vi "fpga_all_example.vi"() -> ()   [LabVIEW 2018]
uses:
  <vilib>/Platform/TimedLoop/XDataNode/timing_clust.ctl
  <vilib>/Platform/TimedLoop/XDataNode/nitl_modes.ctl
  <vilib>/Platform/TimedLoop/XDataNode/wakeup.ctl
  <vilib>/rvi/Emulation/niFpgaGetClockAttributes.vi
  <vilib>/rvi/Emulation/niFpgaSctlEmulationGetInTimedLoop.vi
  <vilib>/rvi/Emulation/niFpgaEmulationReportErrorSimple.vi
  <vilib>/rvi/eio/common/nirviEmuTemplateMethod_errors.vi
  <vilib>/rvi/Emulation/niFpgaCriticalErrorInLSC.vi
  <vilib>/rvi/Emulation/niFpgaProcessEmulError.vi
  lib/Cast-EPICS/cast u64 to u-64-64.vi
  lib/Cast-EPICS/cast u-64-64 to u64.vi
  lib/Cast-EPICS/cast u64 to u-64-0.vi
  lib/Cast-EPICS/cast u-64-0 to u64.vi
  lib/Cast-EPICS/cast u64 to u-64-32.vi
  lib/Cast-EPICS/cast u-64-32 to u64.vi
  lib/Cast-EPICS/cast u64 to s-64-0.vi
  lib/Cast-EPICS/cast s-64-0 to u64.vi
  lib/Cast-EPICS/cast u64 to s-64-64.vi
  lib/Cast-EPICS/cast s-64-64 to u64.vi
  lib/Cast-EPICS/cast u64 to s-64-32.vi
  lib/Cast-EPICS/cast s-64-32 to u64.vi
  <vilib>/eio/EIONode/EIONode.xnode
  <vilib>/Platform/TimedLoop/XDataNode/XDataNode.xnode
  <vilib>/Platform/TimedLoop/XDataNode/XDNodeRunTimeDep.lvlib
  lib/Scaler-EPICS/scaler.lvlib
  lib/Cast-EPICS/fixedpoint-cast.lvlib
panel:
  out "fxp_AnalogOutput3_SCALER2":u64
  out "fxp_AnalogOutput2_SCALER2":u64
  out "fxp_AnalogOutput1_SCALER2":u64
  out "fxp_AnalogOutput0_SCALER2":u64
  in  "fxp_ShiftLeft_SCALER2":u64
  out "fixedpoint_i 1":fxp<+,64,64> format="%.20f"
  out "aifxp 1":u64
  out "fixedpoint_i 2":fxp<+,64,0> format="%#_20g"
  out "aifxp 2":u64
  out "fixedpoint_i 3":fxp<+,64,32> format="%#_20g"
  out "aifxp 3":u64
  out "fixedpoint_i 4":fxp<+/-,64,0> format="%#_20g"
  out "aifxp 4":u64
  out "fixedpoint_i 5":fxp<+/-,64,64> format="%.20f"
  out "aifxp 5":u64
  out "fixedpoint_i 6":fxp<+/-,64,32> format="%#_20g"
  out "aifxp 6":u64
  in  "aofxp 1":u64
  in  "aofxp 2":u64
  in  "aofxp 3":u64
  in  "aofxp 4":u64
  in  "aofxp 5":u64
  in  "aofxp 6":u64
  in  "waveform_u32 2":u32[](array[numeric])=[0, 0, 0]
  out "waveform_u32":u32[](array[numeric])
  out "waveform_u64 2":u64[](array[numeric])
  out "waveform_sgl 2":sgl[](array[numeric]) format="%.2f"
  in  "waveform_u64":u64[](array[numeric])=[0, 0, 0]
  in  "waveform_sgl":sgl[](array[numeric])=[0.0, 0.0, 0.0]
  out "waveform_u16 2":u16[](array[numeric])
  in  "waveform_u16":u16[](array[numeric])=[0, 0, 0]
  out "waveform_u8 2":u8[](array[numeric])
  in  "waveform_u8":u8[](array[numeric])=[0, 0, 0]
  out "waveform_i8 2":i8[](array[numeric])
  in  "waveform_i8":i8[](array[numeric])=[0, 0, 0]
  out "waveform_i16 2":i16[](array[numeric])
  in  "waveform_i16":i16[](array[numeric])=[0, 0, 0]
  out "waveform_i32 2":i32[](array[numeric])
  in  "waveform_i32":i32[](array[numeric])=[0, 0, 0]
  out "waveform_i64 2":i64[](array[numeric])
  in  "waveform_i64":i64[](array[numeric])=[0, 0, 0]
  out "Looptime":u32
  out "AnalogInputs_SCALER2":fxp<+/-,20,5>[](array[numeric])
  in  "PresetValues_SCALER2":u32[](array[numeric])=[0, 0, 0, 0, 0]
  in  "Gate_SCALER2":bool[](array[boolean])=[FALSE, FALSE, FALSE, FALSE, FALSE]
  in  "OneShot_SCALER2":bool
  in  "Enable_SCALER2":bool
  out "Counter_SCALER2":u32[](array[numeric])
  out "Done_SCALER2":bool
  in  "SampleAnalog_SCALER2":bool
  in  "OneShot_SCALER1":bool
  in  "Enable_SCALER1":bool
  in  "Gate_SCALER1":bool[](array[boolean])=[FALSE, FALSE]
  out "Done_SCALER1":bool
  out "Counter_SCALER1":u32[](array[numeric])
  in  "PresetValues_SCALER1":u32[](array[numeric])=[0, 0]
  in  "Pulse_SCALER1":bool[](array[boolean])=[FALSE]
  in  "Mod3/DIO31":bool
  in  "Mod3/DIO30":bool
  in  "Mod3/DIO29":bool
  in  "Mod3/DIO28":bool
  in  "Mod3/DIO27":bool
  in  "Mod3/DIO26":bool
  in  "Mod3/DIO25":bool
  in  "Mod3/DIO24":bool
  in  "Mod3/DIO23":bool
  in  "Mod3/DIO22":bool
  in  "Mod3/DIO21":bool
  in  "Mod3/DIO20":bool
  in  "Mod3/DIO19":bool
  in  "Mod3/DIO18":bool
  in  "Mod3/DIO17":bool
  in  "Mod3/DIO16":bool
  in  "Mod2/DIO0":bool
  in  "Mod2/DIO1":bool
  in  "Mod2/DIO2":bool
  in  "Mod2/DIO3":bool
  in  "Mod1/DIO0":bool
  in  "Mod1/DIO1":bool
  in  "Mod1/DIO2":bool
  in  "Mod1/DIO3":bool
  out "BI":u64
  out "aiMod4/AI3":sgl format="%#_64g"
  out "aiMod4/AI2":sgl format="%#_64g"
  out "aiMod4/AI1":sgl format="%#_64g"
  out "aiMod4/AI0":sgl format="%#_64g"
  in  "aoMod5/AO0":sgl format="%#_64g"
  in  "aoMod5/AO1":sgl format="%#_64g"
  in  "aoMod5/AO2":sgl format="%#_64g"
  in  "aoMod5/AO3":sgl format="%#_64g"
  out "aiMod7/AI3":sgl format="%#_64g"
  out "aiMod7/AI2":sgl format="%#_64g"
  out "aiMod7/AI1":sgl format="%#_64g"
  out "aiMod7/AI0":sgl format="%#_64g"
  out "aiMod8/AI0":sgl format="%#_64g"
  out "aiMod8/AI1":sgl format="%#_64g"
  out "aiMod8/AI2":sgl format="%#_64g"
  out "aiMod8/AI3":sgl format="%#_64g"
  # "Scalers"
  # "Binary outputs"
  # "Analog\nOutput"
  # "Binary\nInput"
  # "Analog Input"
  # "Fixedpoint controls and Indicators"
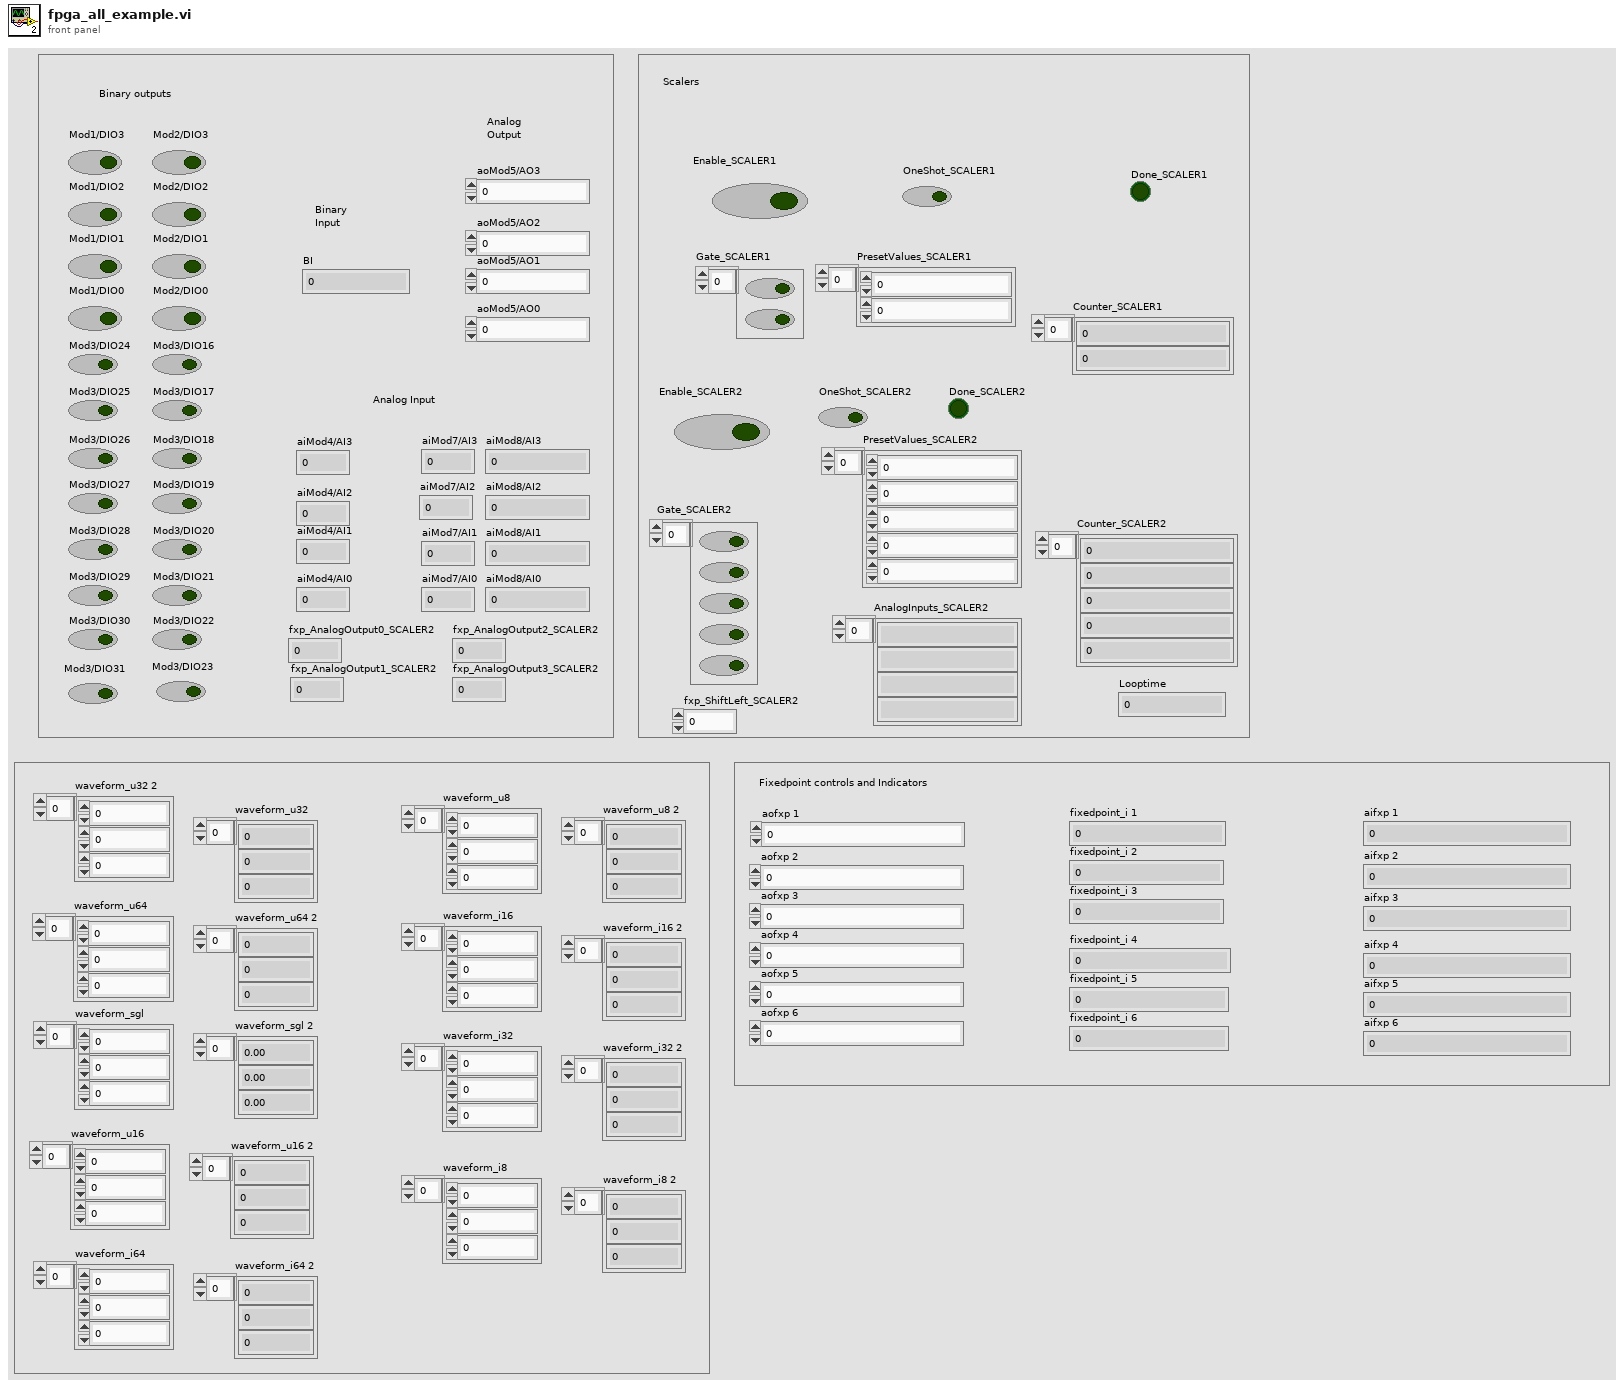
[diagram p1: front panel]
types:
  T1 = typedef "XDNodeRunTimeDep.lvlib/timing_clust.ctl" = cluster{"Expected End [f-1]":u64, "Actual End [f-1]":u64, "Finished Late? [f-1]":bool, "Expected End [i-1]":u64, "Actual End [i-1]":u64, "Finished Late? [i-1]":bool, "Expected Start [i]":u64, "Actual Start [i]":u64, "Expected Start [f]":u64, "Actual Start [f]":u64, "Source Name":string, "Structure Name":string, "Period":i64, "Deadline":i64, "Offset":i64, "Start":i64, "Priority":i32, "Timeout":i32, "Mode":T2, "Wakeup Reason":T3, "Error":errorcluster, "Source Type":string, "Secondary Source Type":string, "Global End Time":u64, "Global Start Time":u64, "Frame Duration":u64, "Iteration Duration":u64, "Assigned CPU":i32, "I/O Scan Engine Mode":u32}
  T2 = typedef "XDNodeRunTimeDep.lvlib/nitl_modes.ctl" = enum32{"No Change", "Process missed periods, maintain original phase", "Discard missed periods, maintain original phase", "Process missed periods, ignore original phase", "Discard missed periods, ignore original phase"}
  T3 = typedef "XDNodeRunTimeDep.lvlib/wakeup.ctl" = enum32{"Normal", "Aborted", "Asynchronous wakeup", "Timing source error", "Timed loop error", "Timeout"}
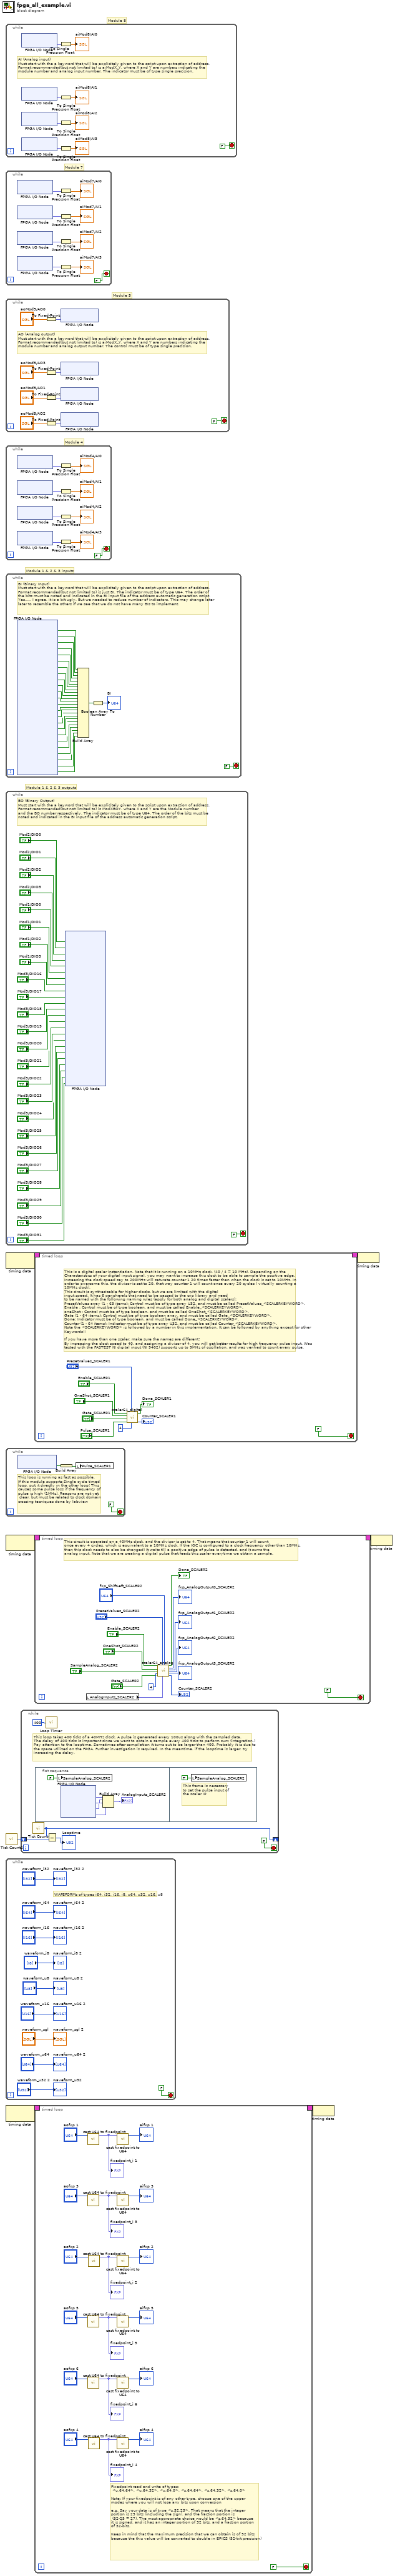
[diagram p0: block diagram]
diagram:
  # "Module 1 & 2 & 3 outputs"
  # "Module 1 & 2 & 3 inputs"
  # "Module 4"
  # "Module 5"
  # "Module 7"
  # "Module 8"
  n1 = while {
    stop <- FALSE stop-if-true
    # "AI (Analog input)\nMust start with the a keyword that will be explicitely given to the script upon extraction of address. \nFormat recommended(but not limited to) is aiModX_Y, where X and Y are numbers indicating the \nmodule number and analog input number. The indicator must be of type single precision."
    n2 = xnode "FPGA I/O Node"() -> ("Mod8/AI0"=w8:fxp<+/-,20,5>)  [unwired: 1 in, 1 out]
    n3 = xnode "FPGA I/O Node"() -> ("Mod8/AI1"=w12:fxp<+/-,20,5>)  [unwired: 1 in, 1 out]
    n4 = xnode "FPGA I/O Node"() -> ("Mod8/AI2"=w10:fxp<+/-,20,5>)  [unwired: 1 in, 1 out]
    n5 = xnode "FPGA I/O Node"() -> ("Mod8/AI3"=w15:fxp<+/-,20,5>)  [unwired: 1 in, 1 out]
    n6 = To Single Precision Float(number=w8) -> (single precision float=→"aiMod8/AI0":sgl)
    n7 = To Single Precision Float(number=w12) -> (single precision float=→"aiMod8/AI1":sgl)
    n8 = To Single Precision Float(number=w10) -> (single precision float=→"aiMod8/AI2":sgl)
    n9 = To Single Precision Float(number=w15) -> (single precision float=→"aiMod8/AI3":sgl)
  }
  n10 = while {
    stop <- FALSE stop-if-true
    n11 = xnode "FPGA I/O Node"() -> ("Mod7/AI0"=w22:fxp<+/-,20,5>)  [unwired: 1 in, 1 out]
    n12 = xnode "FPGA I/O Node"() -> ("Mod7/AI1"=w20:fxp<+/-,20,5>)  [unwired: 1 in, 1 out]
    n13 = xnode "FPGA I/O Node"() -> ("Mod7/AI2"=w18:fxp<+/-,20,5>)  [unwired: 1 in, 1 out]
    n14 = xnode "FPGA I/O Node"() -> ("Mod7/AI3"=w24:fxp<+/-,20,5>)  [unwired: 1 in, 1 out]
    n15 = To Single Precision Float(number=w22) -> (single precision float=→"aiMod7/AI0":sgl)
    n16 = To Single Precision Float(number=w20) -> (single precision float=→"aiMod7/AI1":sgl)
    n17 = To Single Precision Float(number=w18) -> (single precision float=→"aiMod7/AI2":sgl)
    n18 = To Single Precision Float(number=w24) -> (single precision float=→"aiMod7/AI3":sgl)
  }
  n19 = while {
    stop <- FALSE stop-if-true
    # "AO (Analog output)\nMust start with the a keyword that will be explicitely given to the script upon extraction of address. \nFormat recommended(but not limited to) is aiModX_Y, where X and Y are numbers indicating the \nmodule number and analog output number. The control must be of type single precision."
    n20 = To Fixed-Point(number="aoMod5/AO0") -> (fixed-point=w33:fxp<+/-,20,5>)  [unwired: 1 in]
    n21 = To Fixed-Point(number="aoMod5/AO3") -> (fixed-point=w30:fxp<+/-,20,5>)  [unwired: 1 in]
    n22 = To Fixed-Point(number="aoMod5/AO1") -> (fixed-point=w32:fxp<+/-,20,5>)  [unwired: 1 in]
    n23 = To Fixed-Point(number="aoMod5/AO2") -> (fixed-point=w31:fxp<+/-,20,5>)  [unwired: 1 in]
    n24 = xnode "FPGA I/O Node"("Mod5/AO0"=w33) -> ()  [unwired: 1 in, 1 out]
    n25 = xnode "FPGA I/O Node"("Mod5/AO3"=w30) -> ()  [unwired: 1 in, 1 out]
    n26 = xnode "FPGA I/O Node"("Mod5/AO1"=w32) -> ()  [unwired: 1 in, 1 out]
    n27 = xnode "FPGA I/O Node"("Mod5/AO2"=w31) -> ()  [unwired: 1 in, 1 out]
  }
  n28 = while {
    stop <- FALSE stop-if-true
    n29 = xnode "FPGA I/O Node"() -> ("Mod4/AI0"=w40:fxp<+/-,20,5>)  [unwired: 1 in, 1 out]
    n30 = xnode "FPGA I/O Node"() -> ("Mod4/AI1"=w38:fxp<+/-,20,5>)  [unwired: 1 in, 1 out]
    n31 = xnode "FPGA I/O Node"() -> ("Mod4/AI2"=w36:fxp<+/-,20,5>)  [unwired: 1 in, 1 out]
    n32 = xnode "FPGA I/O Node"() -> ("Mod4/AI3"=w42:fxp<+/-,20,5>)  [unwired: 1 in, 1 out]
    n33 = To Single Precision Float(number=w40) -> (single precision float=→"aiMod4/AI0":sgl)
    n34 = To Single Precision Float(number=w38) -> (single precision float=→"aiMod4/AI1":sgl)
    n35 = To Single Precision Float(number=w36) -> (single precision float=→"aiMod4/AI2":sgl)
    n36 = To Single Precision Float(number=w42) -> (single precision float=→"aiMod4/AI3":sgl)
  }
  n37 = while {
    stop <- FALSE stop-if-true
    # "BI (Binary Input)\nMust start with the a keyword that will be explicitely given to the script upon extraction of address. \nFormat recommended(but not limited to) is just BI. The indicator must be of type U64. The order of \nthe bits must be noted and indicated in the BI input file of the address automatic generation script.\nYes...., I agree, it is a bit ugly. But we needed to reduce number of indicators. This may change later\nlater to resemble the others if we see that we do not have many BIs to implement."
    n38 = xnode "FPGA I/O Node"() -> ("Mod3/DIO0"=w70:bool, "Mod3/DIO1"=w69:bool, "Mod3/DIO2"=w66:bool, "Mod3/DIO3"=w65:bool, "Mod3/DIO4"=w64:bool, "Mod3/DIO5"=w63:bool, "Mod3/DIO6"=w62:bool, "Mod3/DIO7"=w61:bool, "Mod3/DIO8"=w60:bool, "Mod3/DIO9"=w59:bool, "Mod3/DIO10"=w58:bool, "Mod3/DIO11"=w57:bool, "Mod3/DIO12"=w56:bool, "Mod3/DIO13"=w55:bool, "Mod3/DIO14"=w54:bool, "Mod3/DIO15"=w53:bool, "Mod1/DIO4"=w51:bool, "Mod1/DIO5"=w50:bool, "Mod1/DIO6"=w49:bool, "Mod1/DIO7"=w48:bool, "Mod2/DIO4"=w47:bool, "Mod2/DIO5"=w46:bool, "Mod2/DIO6"=w45:bool, "Mod2/DIO7"=w44:bool)  [unwired: 24 in, 24 out]
    n39 = Build Array(w70, w69, w66, w65, w64, w63, w62, w61, w60, w59, w58, w57, w56, w55, w54, w53, w51, w50, w49, w48, w47, w46, w45, w44) -> (w52:bool[])
    n40 = Boolean Array To Number(Boolean array=w52) -> (number=→"BI":u64)
  }
  n41 = while {
    stop <- FALSE stop-if-true
    # "BO (Binary Output)\nMust start with the a keyword that will be explicitely given to the script upon extraction of address. \nFormat recommended(but not limited to) is ModXBOY, where X and Y are the Module number \nand the BO number respectively. The indicator must be of type U64. The order of the bits must be \nnoted and indicated in the BI input file of the address automatic generation script."
    n42 = xnode "FPGA I/O Node"("Mod2/DIO0"="Mod2/DIO0", "Mod2/DIO1"="Mod2/DIO1", "Mod2/DIO2"="Mod2/DIO2", "Mod2/DIO3"="Mod2/DIO3", "Mod1/DIO0"="Mod1/DIO0", "Mod1/DIO1"="Mod1/DIO1", "Mod1/DIO2"="Mod1/DIO2", "Mod1/DIO3"="Mod1/DIO3", "Mod3/DIO16"="Mod3/DIO16", "Mod3/DIO17"="Mod3/DIO17", "Mod3/DIO18"="Mod3/DIO18", "Mod3/DIO19"="Mod3/DIO19", "Mod3/DIO20"="Mod3/DIO20", "Mod3/DIO21"="Mod3/DIO21", "Mod3/DIO22"="Mod3/DIO22", "Mod3/DIO23"="Mod3/DIO23", "Mod3/DIO24"="Mod3/DIO24", "Mod3/DIO25"="Mod3/DIO25", "Mod3/DIO26"="Mod3/DIO26", "Mod3/DIO27"="Mod3/DIO27", "Mod3/DIO28"="Mod3/DIO28", "Mod3/DIO29"="Mod3/DIO29", "Mod3/DIO30"="Mod3/DIO30", "Mod3/DIO31"="Mod3/DIO31") -> ()  [unwired: 24 in, 24 out]
  }
  n43 = node-c288() -> (w7:T1)  [unwired: 1 in]
  n44 = while {
    stop <- FALSE stop-if-true
    # "This loop is running as fast as possible. \nIf this module supports Single cycle timed\nloop, put it directly in the other loop! This\ncauses some pulse loss if the frequency of \npulse is high (1MHz). Reasons are not yet\n clear, but must be related to clock domain\ncrossing tecniques done by labview"
    n45 = xnode "FPGA I/O Node"() -> ("Mod2/DIO0"=w98:bool)  [unwired: 1 in, 1 out]
    n46 = Build Array(w98) -> (w97:bool[])
    n47 = local write "Pulse_SCALER1"(w97) -> ()
  }
  n48 = node-c288() -> (w5:T1)  [unwired: 1 in]
  n49 = call "Tick Count2"() -> ("Tick Count(Ticks)"=w3:u32)
  n50 = while {
    stop <- FALSE stop-if-true
    # "WAFEFORMs of types i64, i32, i16, i8, u64, u32, u16, u8"
    "waveform_u32" <- "waveform_u32 2"
    "waveform_u64 2" <- "waveform_u64"
    "waveform_sgl 2" <- "waveform_sgl"
    "waveform_u16 2" <- "waveform_u16"
    "waveform_u8 2" <- "waveform_u8"
    "waveform_i8 2" <- "waveform_i8"
    "waveform_i16 2" <- "waveform_i16"
    "waveform_i32 2" <- "waveform_i32"
    "waveform_i64 2" <- "waveform_i64"
  }
  n51 = node-c288() -> (w2:T1)  [unwired: 1 in]
  n52 = while {
    shift-right: [w110] -> _
    shift-left: w3 -> [w111]
    stop <- FALSE stop-if-true
    # "This loop takes 400 ticks of a 40MHz clock. A pulse is generated every 100us along with the sampled data. \nThe delay of 400 ticks is important since we want to obtain a sample every 400 ticks to perform sum (integration.)\nPay attention to the looptime. Sometimes after compilation it turns out to be larger than 400. Probably it is due to \nthe space utilized on the FPGA. Further investigation is required. In the meantime, if the looptime is larger, try\nincreasing the delay."
    n53 = call "Tick Count"() -> ("Tick Count(Ticks)"=w110:u32)
    n54 = flat-sequence {
      frame #0 {
        n55 = local write "SampleAnalog_SCALER2"(FALSE) -> ()
        n56 = xnode "FPGA I/O Node"() -> ("Mod4/AI0"=w119:fxp<+/-,20,5>, "Mod4/AI1"=w116:fxp<+/-,20,5>, "Mod4/AI2"=w115:fxp<+/-,20,5>, "Mod4/AI3"=w114:fxp<+/-,20,5>)  [unwired: 4 in, 4 out]
        n57 = Build Array(w119, w116, w115, w114) -> (→"AnalogInputs_SCALER2":fxp<+/-,20,5>[])
      }
      frame #1 {
        # "This frame is necessary to set the pulse input of the scaler IP"
        n58 = local write "SampleAnalog_SCALER2"(TRUE ("sample")) -> ()
      }
    }
    n59 = call "Loop Timer"("Count(Ticks)"=i16 400) -> ()  [unwired: 1 out]
    n60 = Subtract(x=w110, y=w111) -> (x-y=→"Looptime":u32)
  }
  n61 = timed-loop {
    timing: w7 -> [_]
    timing-out: [_] -> w6
    stop <- FALSE stop-if-true
    # "This is a digital scaler instantiation. Note that it is running on a 10MHz clock. (40 / 4 = 10 MHz). Depending on the \nCharacteristics of your digital input signal, you may want to increase this clock to be able to sample the positive edge.\nIncreasing the clock speed say to 200MHz will saturate counter 1 20 times faster than when the clock is set to 10MHz. In\norder to overcome this, the divisor is set to 20, that way counter 1 will count once every 20 cycles ( virtually counting a \n10MHz clock).\nThis circuit is synthesizable for higher clocks, but we are limited with the digital \ninput speed. It has 6 peripherals that need to be passed to the crio library and need \nto be named with the following naming rules (apply for both analog and digital scalers): \nPresetValues array (1 - 63 items): Control must be of type array U32, and must be called PresetValues_<SCALERKEYWORD>. \nEnable : Control must be of type boolean, and must be called Enable_<SCALERKEYWORD>. \noneShot : Control must be of type boolean, and must be called OneShot_<SCALERKEYWORD>. \nGate (1 - 64 items): Control must be of type boolean array, and must be called Gate_<SCALERKEYWORD>. \nDone: Indicator must be of type boolean, and must be called Done_<SCALERKEYWORD>. \nCounter (1 - 64 items): Indicator must be of type array U32, and must be called Counter_<SCALERKEYWORD>. \nNote the <SCALERKEYWORD> is followed by a number in this implementation. It can be followed by anything except for other Keywords!!\n\nIf you have more than one scaler, make sure the names are different!\nBy increasing the clock speed to 40, and assigning a divisor of 4, you will get better results for high frequency pulse input. Was tested with the FASTEST NI digital input (NI 9402) supports up to 9MHz of oscillation, and was verified to count every pulse."
    n62 = call "scaler64_digital.vi"("divisor_SCALER"=i16 4, "PresetValues_SCALER"="PresetValues_SCALER1", "Pulse_SCALER"="Pulse_SCALER1", "Gate_SCALER"="Gate_SCALER1", "OneShot_SCALER"="OneShot_SCALER1", "Enable_SCALER"="Enable_SCALER1") -> ("Counter_SCALER"=→"Counter_SCALER1":u32[], "Done_SCALER"=→"Done_SCALER1":bool)  [unwired: 4 in]
  }
  n63 = timed-loop {
    timing: w5 -> [_]
    timing-out: [_] -> w4
    stop <- FALSE stop-if-true
    # "This circuit is operated on a 40MHz clock, and the divisor is set to 4. That means that counter 1 will count \nonce every 4 cycles, which is equivalent to a 10MHz clock. If the IOC is configured to a clock frequency other than 10MHz, \nthen this clock needs to also be changed! It waits till a positive edge of pulse is detected, and it sums the\nanalog input. Note that we are creating a digital pulse that feeds this scaler everytime we obtain a sample."
    n64 = local read "AnalogInputs_SCALER2"() -> (w140:fxp<+/-,20,5>[])
    n65 = call "scaler64_analog.vi"("Enable_SCALER"="Enable_SCALER2", "OneShot_SCALER"="OneShot_SCALER2", "SampleAnalog_SCALER"="SampleAnalog_SCALER2", "Gate_SCALER"="Gate_SCALER2", "PresetValues_SCALER"="PresetValues_SCALER2", "AnalogInputs_SCALER"=w140, "fxp_ShiftLeft_SCALER"="fxp_ShiftLeft_SCALER2", "divisor_SCALER"=i16 4) -> ("Done_SCALER"=→"Done_SCALER2":bool, "fxp_AnalogOutput0_SCALER"=→"fxp_AnalogOutput0_SCALER2":u64, "fxp_AnalogOutput1_SCALER"=→"fxp_AnalogOutput1_SCALER2":u64, "fxp_AnalogOutput2_SCALER"=→"fxp_AnalogOutput2_SCALER2":u64, "fxp_AnalogOutput3_SCALER"=→"fxp_AnalogOutput3_SCALER2":u64, "Counter_SCALER"=→"Counter_SCALER2":u32[])  [unwired: 6 in]
  }
  n66 = timed-loop {
    timing: w2 -> [_]
    timing-out: [_] -> w1
    stop <- FALSE stop-if-true
    # "Fixedpoint read and write of types:\n <u,64,64>, <u,64,32>, <u,64,0>, <s,64,64>, <s,64,32>, <s,64,0>\n\nNote: If your fixedpoint is of any other type, choose one of the upper\nmodes where you will not lose any bits upon conversion\n\ne.g. Say your data is of type <s,52,25>. That means that the integer\nportion is 25 bits (including the sign), and the fraction portion is\n (52-25 = 27). The most appropriate choice would be <s,64,32> because\nit is signed, and it has an integer portion of 32 bits, and a fraction portion\nof 32-bits. \n\nKeep in mind that the maximum precision that we can obtain is of 52 bits\nbecause the this value will be converted to double in EPICS (52-bit precision)"
    n67 = call-poly "cast U64 to fixedpoint.vi"("aofxp"="aofxp 1") -> ("fixedpoint_o"=w160:fxp<+,64,64>)  [unwired: 10 in]
    "fixedpoint_i 1" <- w160
    n68 = call-poly "cast U64 to fixedpoint.vi"("aofxp"="aofxp 3") -> ("fixedpoint_o"=w155:fxp<+,64,32>)  [unwired: 10 in]
    "fixedpoint_i 3" <- w155
    n69 = call-poly "cast U64 to fixedpoint.vi"("aofxp"="aofxp 5") -> ("fixedpoint_o"=w157:fxp<+/-,64,64>)  [unwired: 10 in]
    "fixedpoint_i 5" <- w157
    n70 = call-poly "cast U64 to fixedpoint.vi"("aofxp"="aofxp 6") -> ("fixedpoint_o"=w158:fxp<+/-,64,32>)  [unwired: 10 in]
    "fixedpoint_i 6" <- w158
    n71 = call-poly "cast U64 to fixedpoint.vi"("aofxp"="aofxp 2") -> ("fixedpoint_o"=w156:fxp<+,64,0>)  [unwired: 10 in]
    "fixedpoint_i 2" <- w156
    n72 = call-poly "cast U64 to fixedpoint.vi"("aofxp"="aofxp 4") -> ("fixedpoint_o"=w159:fxp<+/-,64,0>)  [unwired: 10 in]
    "fixedpoint_i 4" <- w159
    n73 = call-poly "cast fixedpoint to U64.vi"("fixedpoint_i"=w160) -> ("aifxp"=→"aifxp 1":u64)  [unwired: 10 in]
    n74 = call-poly "cast fixedpoint to U64.vi"("fixedpoint_i"=w155) -> ("aifxp"=→"aifxp 3":u64)  [unwired: 10 in]
    n75 = call-poly "cast fixedpoint to U64.vi"("fixedpoint_i"=w156) -> ("aifxp"=→"aifxp 2":u64)  [unwired: 10 in]
    n76 = call-poly "cast fixedpoint to U64.vi"("fixedpoint_i"=w157) -> ("aifxp"=→"aifxp 5":u64)  [unwired: 10 in]
    n77 = call-poly "cast fixedpoint to U64.vi"("fixedpoint_i"=w158) -> ("aifxp"=→"aifxp 6":u64)  [unwired: 10 in]
    n78 = call-poly "cast fixedpoint to U64.vi"("fixedpoint_i"=w159) -> ("aifxp"=→"aifxp 4":u64)  [unwired: 10 in]
  }
  n79 = node-c288(w1) -> ()
  n80 = node-c288(w6) -> ()
  n81 = node-c288(w4) -> ()
